vi "Picture Display Global.vi"() -> ()   [LabVIEW 2020]
panel:
  in  "Camera4":string
  in  "Camera3":string
  in  "Camera2":string
  in  "Camera1":string
  out "Image 4 Time":timestamp
  out "Image 2 Time":timestamp
  out "Image 1 Time":timestamp
  out "Image 3 Time":timestamp
  out "Image 4":T1(plugin-control)
  out "Image 3":T1(plugin-control)
  out "Image 2":T1(plugin-control)
  out "Image 1":T1(plugin-control)
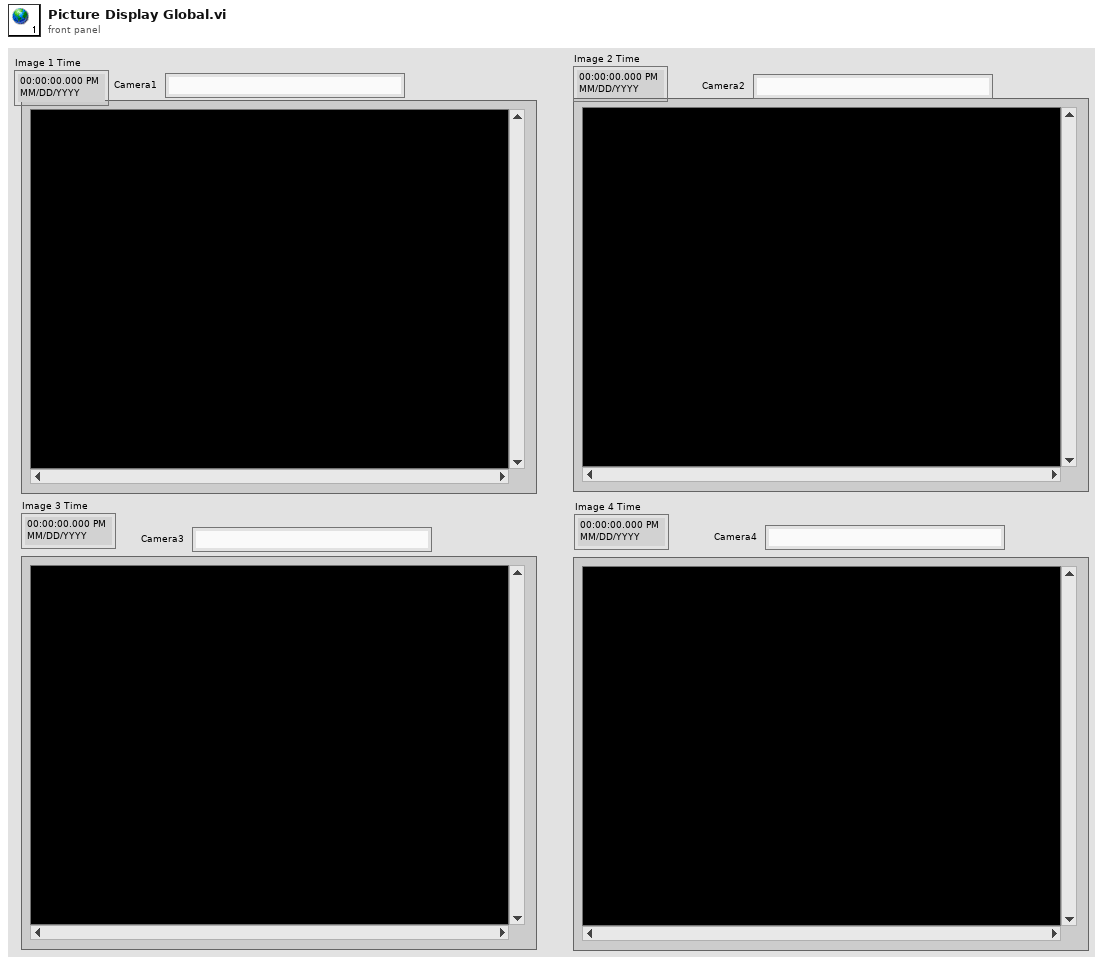
[diagram p1: front panel]
types:
  T1 = typedef "IMAQ Image.ctl" = refnum<image>
diagram:
